vi "Connect.vi"(8 "error in (no error)":errorcluster, 10 "Params":variant, 11 "Switching in":refnum<class "PIPX40 Relay.lvclass">) -> (0 "error out":errorcluster, 3 "Switching out":refnum<class "PIPX40 Relay.lvclass">)   [LabVIEW 2020, in "Pickering.lvlib" / "PIPX40 Relay.lvclass"]
uses:
  PIPX40 Relay.lvclass
  D:/WSGitHub/RTFWK/Realization/PIPX40 Base/PIPX40 Base.lvclass
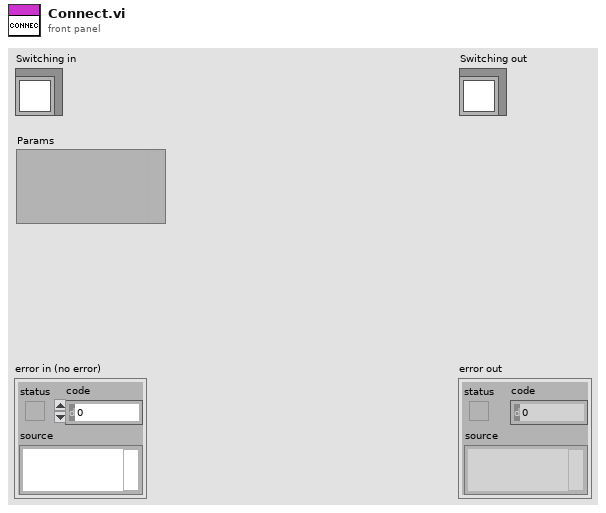
[diagram p1: front panel]
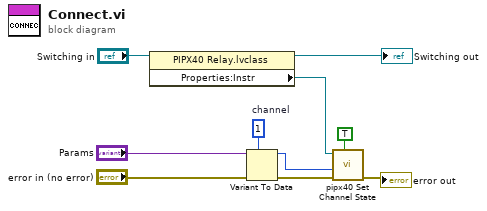
[diagram p0: block diagram]
diagram:
  w5 = u32 1  # channel
  n1 = property class="PIPX40 Relay.lvclass"(reference="Switching in") -> (reference out=→"Switching out":refnum<class "PIPX40 Relay.lvclass">, "Properties:Instr"=w2:refnum<visa-resource-name>)  [unwired: 1 in, 1 out]
  n2 = Variant To Data(error in="error in (no error)", type=w5, Variant="Params") -> (data=w1:u32, error out=w8:errorcluster)
  n3 = call <instrlib>:"pipx40 Set Channel State.vi"("action"=TRUE, "error in (no error)"=w8, "channel number"=w1, "instrument handle"=w2) -> ("error out"=→"error out":errorcluster)  [unwired: 6 in, 1 out]
